vi "List Sensors.vi"(8 "error in (no error)":errorcluster, 11 "Edit Test Channel Model in":refnum<class "Edit Test Channel Model.lvclass">) -> (0 "error out":errorcluster, 3 "Edit Test Channel Model out":refnum<class "Edit Test Channel Model.lvclass">)   [LabVIEW 2013, in "Edit Test Channel Model.lvlib" / "Edit Test Channel Model.lvclass"]
uses:
  Edit Test Channel Model.lvclass
  Edit Test Channel Model.lvclass/Edit Test Channel Model.ctl
  Common/File IO/File IO.lvlib
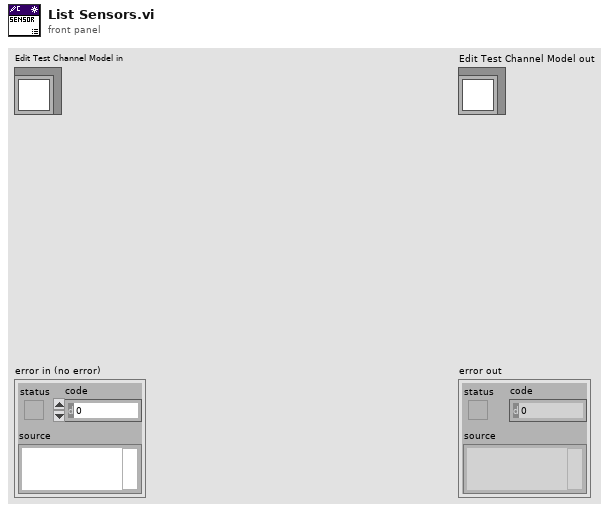
[diagram p1: front panel]
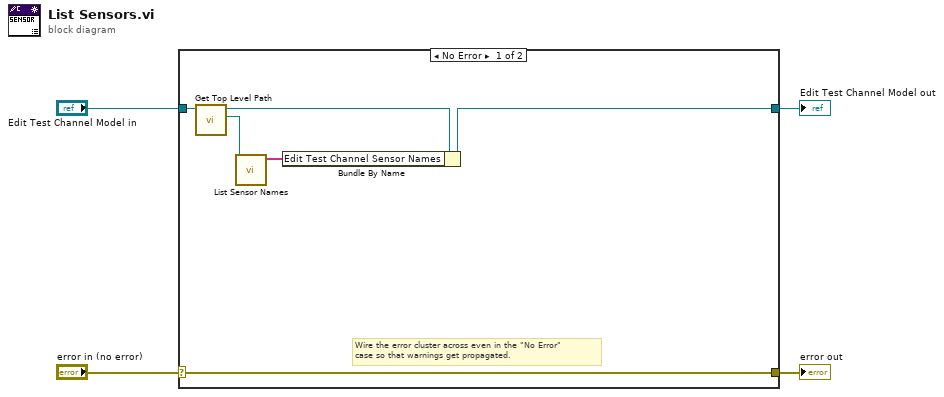
[diagram p0: block diagram]
diagram:
  n1 = case shown="No Error" "error in (no error)" {
    selector: "error in (no error)" -> [w10 w12]
    tunnel: [w10 w12] -> w3
    tunnel: [w7 w11] -> w1
    tunnel: "Edit Test Channel Model in" -> [w8 w11]
    frame No Error {
      # "Wire the error cluster across even in the \"No Error\"\ncase so that warnings get propagated."
      n2 = call-dynamic "Get Top Level Path.vi"("Abstract Model in"=w8) -> ("Top Level Path"=w5:path, "Abstract Model out"=w6:refnum<class "Edit Test Channel Model.lvclass">)  [unwired: 8 in, 1 out]
      n3 = call "List Sensor Names.vi"("Top Level Path"=w5) -> ("Sensor Names"=w9:string[])  [unwired: 10 in]
      n4 = Bundle By Name(cluster=w6, "Edit Test Channel Sensor Names"=w9) -> (w7:refnum<class "Edit Test Channel Model.lvclass">)
    }
    frame Error {
    }
  }
  "error out" <- w3
  "Edit Test Channel Model out" <- w1
